vi "NewFile.vi"(8 "error in (no error)":errorcluster, 9 "data flow":T13, 10 "data event":T17, 11 "config":T22) -> (0 "error out":errorcluster, 2 "data event config":T17, 3 "data event":T1, 4 "registry":T9, 5 "save waveforms":bool)   [LabVIEW 2017, in "DataEventCreator.lvlib"]
uses:
  <vilib>/addons/InsightCM/Devices/Shared/Common/DataEventCreator/DataEventCreator.lvlib
  <vilib>/addons/InsightCM/MessageBus/Base/controls/KeyValuePair.ctl
  <vilib>/addons/InsightCM/MessageBus/Base/controls/DataEvent.ctl
  <vilib>/addons/InsightCM/MessageBus/Base/controls/DataSetMetadata.ctl
  <vilib>/addons/InsightCM/Devices/Shared/Common/DataEvent/controls/DataSet.ctl
  <vilib>/addons/InsightCM/Devices/Shared/Common/DataEvent/DataEvent.lvlib
  <vilib>/addons/InsightCM/MessageBus/Base/controls/TrendPoint.ctl
  <vilib>/addons/InsightCM/Devices/Shared/Common/DataEvent/controls/Event.ctl
  <vilib>/addons/InsightCM/SRP/SRP.lvlib
  <vilib>/addons/InsightCM/Devices/Shared/Common/DataEvent/controls/DataSetType.ctl
  <vilib>/addons/InsightCM/Devices/Shared/Cms/CmsDataEventCreator/controls/DataSetRegistry.ctl
  <vilib>/addons/InsightCM/Devices/Shared/Cms/CmsDataEventCreator/CmsDataEventCreator.lvlib
  <vilib>/addons/InsightCM/Devices/Shared/Common/DataEventCreator/controls/Registry_Trend.ctl
  <vilib>/addons/InsightCM/Devices/Shared/Cms/CmsDataEventCreator/controls/GroupRegistry.ctl
  <vilib>/addons/InsightCM/MessageBus/Base/controls/TrendAlarmTransition.ctl
  <vilib>/addons/InsightCM/MessageBus/Base/controls/TrendAlarmUpdate.ctl
  <vilib>/addons/InsightCM/Utilities/DataAccessors/controls/wfmSGL_DVR.ctl
  <vilib>/addons/PointValueMap/controls/PointMap.ctl
  <vilib>/addons/PointValueMap/PointValueMap.lvlib
  <vilib>/addons/InsightCM/Devices/Shared/Cms/CmsDataEventCreator/controls/AcqParams.ctl
  <vilib>/addons/InsightCM/Devices/Shared/Cms/CmsDataEventCreator/controls/DataEventConfig.ctl
  <vilib>/addons/InsightCM/Devices/Shared/Common/DataAccumulator/controls/accumulationType.ctl
  <vilib>/addons/InsightCM/Devices/Shared/Common/DataAccumulator/DataAccumulator.lvlib
  <vilib>/addons/InsightCM/Devices/Shared/Common/DVRBuffer/controls/BufferLocation.ctl
  <vilib>/addons/InsightCM/Devices/Shared/Common/DVRBuffer/DVRBuffer.lvlib
  <vilib>/addons/InsightCM/Devices/Shared/Common/DataAccumulator/controls/AccumulationSettings.ctl
  <vilib>/addons/InsightCM/Devices/Shared/Common/DataFlow/controls/Data.ctl
  <vilib>/addons/InsightCM/Devices/Shared/Common/DataFlow/DataFlow.lvlib
  <vilib>/addons/InsightCM/Devices/Shared/Cms/CmsDataEventCreator/controls/config.ctl
  <vilib>/addons/InsightCM/Devices/Shared/Common/DataFlow/controls/Type.ctl
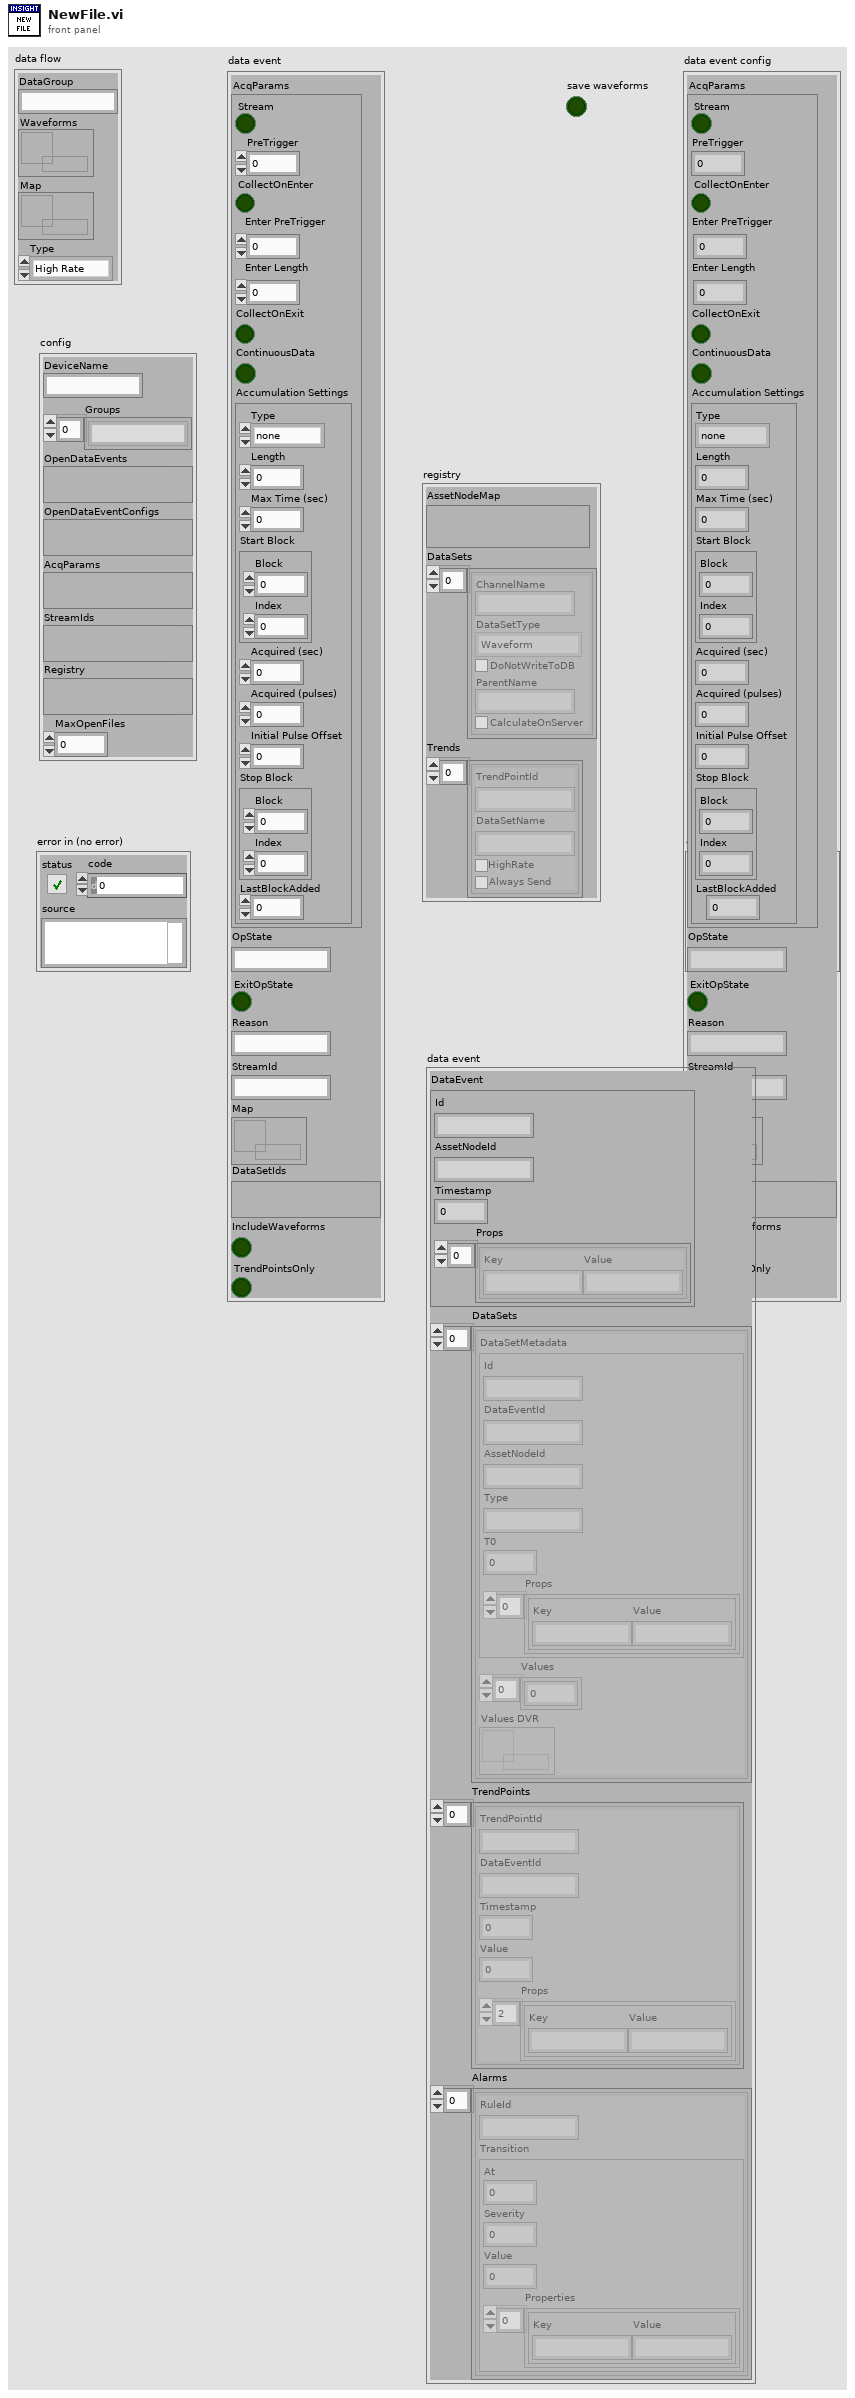
[diagram p1: front panel]
types:
  T1 = typedef "DataEvent.lvlib/Event.ctl" = cluster{"DataEvent":T2, "DataSets":T4[], "TrendPoints":T6[], "Alarms":T7[]}
  T2 = typedef "DataEvent.ctl" = cluster{"Id":string, "AssetNodeId":string, "Timestamp":i64, "Props":T3[]}
  T3 = typedef "KeyValuePair.ctl" = cluster{"Key":string, "Value":string}
  T4 = typedef "DataEvent.lvlib/DataSet.ctl" = cluster{"DataSetMetadata":T5, "Values":sgl[], "Values DVR":refnum<data-value>}
  T5 = typedef "DataSetMetadata.ctl" = cluster{"Id":string, "DataEventId":string, "AssetNodeId":string, "Type":string, "T0":i64, "Props":T3[]}
  T6 = typedef "TrendPoint.ctl" = cluster{"TrendPointId":string, "DataEventId":string, "Timestamp":i64, "Value":dbl, "Props":T3[]}
  T7 = typedef "TrendAlarmUpdate.ctl" = cluster{"RuleId":string, "Transition":T8}
  T8 = typedef "TrendAlarmTransition.ctl" = cluster{"At":i64, "Severity":i32, "Value":dbl, "Properties":T3[]}
  T9 = typedef "CmsDataEventCreator.lvlib/GroupRegistry.ctl" = cluster{"AssetNodeMap":variant, "DataSets":T10[], "Trends":T12[]}
  T10 = typedef "CmsDataEventCreator.lvlib/DataSetRegistry.ctl" = cluster{"ChannelName":string, "DataSetType":T11, "DoNotWriteToDB":bool, "ParentName":string, "CalculateOnServer":bool}
  T11 = typedef "DataEvent.lvlib/DataSetType.ctl" = enum16{"Waveform", "SpeedProfile", "ThermalImage", "EmsaSweep"}
  T12 = typedef "DataEventCreator.lvlib/Registry_Trend.ctl" = cluster{"TrendPointId":string, "DataSetName":string, "HighRate":bool, "Always Send":bool}
  T13 = typedef "DataFlow.lvlib/Data.ctl" = cluster{"DataGroup":string, "Waveforms":T14, "Map":T15, "Type":T16}
  T14 = typedef "wfmSGL_DVR.ctl" = refnum<data-value>
  T15 = typedef "PointValueMap.lvlib/PointMap.ctl" = refnum<data-value>
  T16 = typedef "DataFlow.lvlib/Type.ctl" = enum16{"High Rate", "Low Rate", "Burst Mode"}
  T17 = typedef "CmsDataEventCreator.lvlib/DataEventConfig.ctl" = cluster{"AcqParams":T18, "OpState":string, "ExitOpState":bool, "Reason":string, "StreamId":string, "Map":T15, "DataSetIds":variant, "IncludeWaveforms":bool, "TrendPointsOnly":bool}
  T18 = typedef "CmsDataEventCreator.lvlib/AcqParams.ctl" = cluster{"Stream":bool, "PreTrigger":i32, "CollectOnEnter":bool, "Enter PreTrigger":i32, "Enter Length":dbl, "CollectOnExit":bool, "ContinuousData":bool, "Accumulation Settings":T19}
  T19 = typedef "DataAccumulator.lvlib/AccumulationSettings.ctl" = cluster{"Type":T20, "Length":dbl, "Max Time (sec)":dbl, "Start Block":T21, "Acquired (sec)":dbl, "Acquired (pulses)":i32, "Initial Pulse Offset":dbl, "Stop Block":T21, "LastBlockAdded":u32}
  T20 = typedef "DataAccumulator.lvlib/accumulationType.ctl" = enum16{"none", "seconds", "revolutions"}
  T21 = typedef "DVRBuffer.lvlib/BufferLocation.ctl" = cluster{"Block":u32, "Index":i32}
  T22 = typedef "CmsDataEventCreator.lvlib/config.ctl" = cluster{"DeviceName":string, "Groups":string[], "OpenDataEvents":variant, "OpenDataEventConfigs":variant, "AcqParams":variant, "StreamIds":variant, "Registry":variant, "MaxOpenFiles":i32}
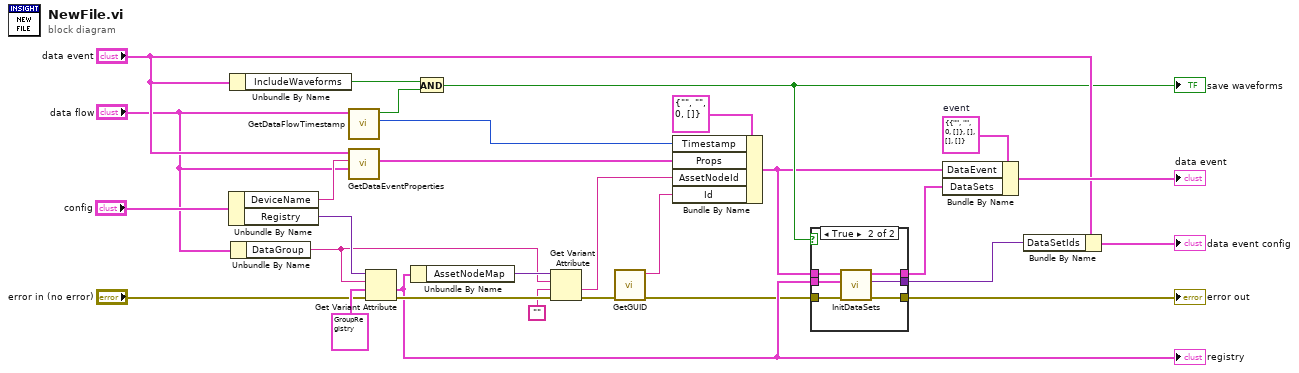
[diagram p0: block diagram]
diagram:
  w26 = T1 {"DataEvent"={"Id"="", "AssetNodeId"="", "Timestamp"=0, "Props"=[]}, "DataSets"=[], "TrendPoints"=[], "Alarms"=[]}  # event
  n1 = Unbundle By Name("config") -> ("DeviceName"=w11:string, "Registry"=w29:variant)
  n2 = Unbundle By Name("data event") -> ("IncludeWaveforms"=w12:bool)
  n3 = Unbundle By Name("data flow") -> ("DataGroup"=w10:string)
  n4 = call <vilib>:"GetDataFlowTimestamp.vi"("data"="data flow") -> ("unix timestamp"=w9:i64, "has waveforms"=w13:bool)  [unwired: 9 in]
  n5 = call <vilib>:"GetDataEventProperties.vi"("data"="data flow", "device name"=w11, "data event"="data event") -> ("data event properties"=w15:T3[])  [unwired: 8 in]
  n6 = Get Variant Attribute(Variant=w29, name=w10, default value (empty Variant)=T9 {"AssetNodeMap"=variant, "DataSets"=[], "Trends"=[]} ("Data Group Registry"), error in="error in (no error)") -> (value=w6:T9, error out=w22:errorcluster)  [unwired: 2 out]
  "registry" <- w6
  n7 = Unbundle By Name(w6) -> ("AssetNodeMap"=w23:variant)
  n8 = And(x=w12, y=w13) -> (x .and. y?=w7:bool)
  "save waveforms" <- w7
  n9 = Get Variant Attribute(Variant=w23, name=w10, default value (empty Variant)="", error in=w22) -> (value=w19:string, error out=w16:errorcluster)  [unwired: 2 out]
  n10 = call <vilib>:"GetGUID.vi"("error in (no error)"=w16) -> ("error out"=w5:errorcluster, "GUID"=w18:string)  [unwired: 9 in]
  n11 = Bundle By Name(cluster=T2 {"Id"="", "AssetNodeId"="", "Timestamp"=0, "Props"=[]} ("DataEvent"), "Timestamp"=w9, "Props"=w15, "AssetNodeId"=w19, "Id"=w18) -> (w2:T2)
  n12 = case shown="True" w7 {
    tunnel: w6 -> [_ w32]
    tunnel: w5 -> [w30 w36]
    tunnel: [_ w35] -> w4
    tunnel: [w30 w34] -> w1
    tunnel: [_ w33] -> w3
    tunnel: w2 -> [_ w31]
    frame False {
    }
    frame True {
      n13 = call <vilib>:"InitDataSets.vi"("error in (no error)"=w36, "registry"=w32, "dataevent"=w31) -> ("error out"=w34:errorcluster, "datasetIds"=w35:variant, "datasets"=w33:T4[])  [unwired: 6 in]
    }
  }
  "error out" <- w1
  n14 = Bundle By Name(cluster=w26, "DataEvent"=w2, "DataSets"=w3) -> (→"data event":T1)
  n15 = Bundle By Name(cluster="data event", "DataSetIds"=w4) -> (→"data event config":T17)
